vi "Execute.vi"(8 "error in (no error)":errorcluster, 10 "System In":refnum<class "abs_System.lvclass">, 11 "Node in":refnum<class "Test Numeric.lvclass">) -> (0 "error out":errorcluster, 1 "Status":T1, 2 "System Out":refnum<class "abs_System.lvclass">, 3 "Node out":refnum<class "Test Numeric.lvclass">)   [LabVIEW 2021, in "BT.lvlib" / "Test Numeric.lvclass"]
uses:
  Test Numeric.lvclass
  C:/Users/Tim/Documents/LabVIEW/2021/Behaviour Tree/Source/abs_Type Leaf/abs_Type Leaf.lvclass
  abs_Node/Status.ctl
  abs_System/abs_System.lvclass
  GitHub/LV_Abstract/Source/Abs_Types/Double Float/Abs_Double Float.lvclass
  abs_Type Leaf/abs_Type Leaf.lvclass/abs_Type Leaf.ctl
  Test Numeric.lvclass/Test Numeric.ctl
  abs_Type Leaf/Properties/Read Value Class.vi
  Properties/Read Lower Limit.vi
  Properties/Read Upper Limit.vi
  Properties/Read Limit Test Type.vi
  GitHub/LV_Abstract/Source/Functions/Compare/Support/Greater/DBL/Method.vi
  GitHub/LV_Abstract/Source/Functions/Compare/Support/Less/DBL/Method.vi
  GitHub/LV_Abstract/Source/Functions/Compare/Support/Greater Equal/DBL/Method.vi
  GitHub/LV_Abstract/Source/Functions/Compare/Support/Less Equal/DBL/Method.vi
  GitHub/LV_Abstract/Source/Functions/Logic/Support/AND/Bool/Method.vi
  GitHub/LV_Abstract/Source/Functions/Logic/Support/OR/Bool/Method.vi
  GitHub/LV_Abstract/Source/Abs_Types/Type/Abs_Type.lvclass
  GitHub/LV_Abstract/Source/Abs_Types/Numeric/Abs_Numeric.lvclass
  abs_Type Leaf/abs_Type Leaf.lvclass
  GitHub/LV_Abstract/Source/Abs_Types/Boolean/Abs_Boolean.lvclass
  GitHub/LV_Abstract/Source/Functions/Compare/Support/Equal/DBL/Method.vi
  GitHub/LV_Abstract/Source/Functions/Compare/Support/Not Equal/DBL/Method.vi
  abs_Node/abs_Node.lvclass
  GitHub/LV_Abstract/Source/Functions/Compare/Support/Greater/DBL/Greater_DBL.lvclass
  GitHub/LV_Abstract/Source/Functions/Compare/Support/Less/DBL/Less_DBL.lvclass
  GitHub/LV_Abstract/Source/Functions/Compare/Support/Greater Equal/DBL/Greater Equal_DBL.lvclass
  GitHub/LV_Abstract/Source/Functions/Compare/Support/Less Equal/DBL/Less Equal_DBL.lvclass
  GitHub/LV_Abstract/Source/Functions/Logic/Support/AND/Bool/AND_Bool.lvclass
  GitHub/LV_Abstract/Source/Functions/Logic/Support/OR/Bool/OR_Bool.lvclass
  GitHub/LV_Abstract/Source/Functions/Conversion/Support/DBL/ConvertTo_DBL.lvclass
  C:/Users/Tim/Documents/GitHub/LV_Abstract/Source/Abs_Types/Double Float/Abs_Double Float.lvclass
  C:/Users/Tim/Documents/GitHub/LV_Abstract/Source/Abs_Types/Floating Point/Abs_Floating Point.lvclass
  C:/Users/Tim/Documents/GitHub/LV_Abstract/Source/Abs_Types/Numeric/Abs_Numeric.lvclass
  C:/Users/Tim/Documents/GitHub/LV_Abstract/Source/Abs_Types/Value/Abs_Value.lvclass
  C:/Users/Tim/Documents/GitHub/LV_Abstract/Source/Abs_Types/Type/Abs_Type.lvclass
  C:/Users/Tim/Documents/GitHub/LV_Abstract/Source/Functions/Conversion/Support/DBL/ConvertTo_DBL.lvclass
  GitHub/LV_Abstract/Source/Functions/Compare/Support/Equal/DBL/Equal_DBL.lvclass
  GitHub/LV_Abstract/Source/Functions/Compare/Support/Not Equal/DBL/Not Equal_DBL.lvclass
  GitHub/LV_Abstract/Source/Functions/Math/Support/Add/DBL/Method.vi
  GitHub/LV_Abstract/Source/Functions/Math/Support/Add/DBL/Add_DBL.lvclass
  GitHub/LV_Abstract/Source/Functions/Math/Support/Subtract/DBL/Method.vi
  GitHub/LV_Abstract/Source/Functions/Math/Support/Subtract/DBL/Subtract_DBL.lvclass
  GitHub/LV_Abstract/Source/Functions/Conversion/Support/DBL/Method.vi
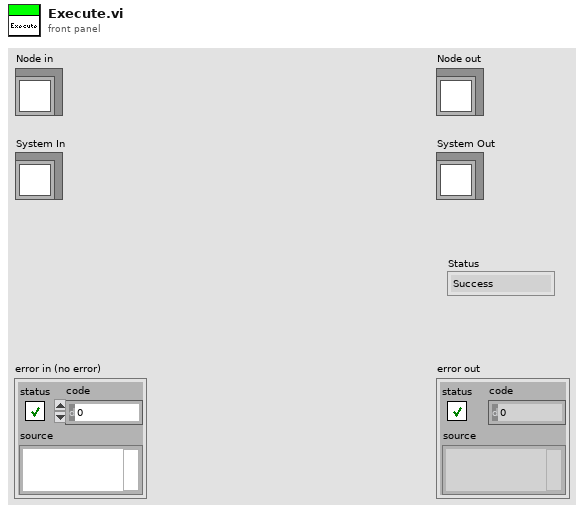
[diagram p1: front panel]
types:
  T1 = typedef "BT.lvlib/abs_Node.lvclass/Status.ctl" = enum16{"Success", "Failure", "Running"}
  T2 = typedef "BT.lvlib/Limit Test Type.ctl" = enum16{"x == Lo", "x != Lo", "x > Lo", "x < Lo", "x >= Lo", "x <= Lo", "Lo > x < Hi", "Lo >= x <= Hi", "Lo >= x < Hi", "Lo > x <= Hi", "Lo < x > Hi", "Lo <= x >= Hi", "Lo <= x > Hi", "Lo < x >= Hi", "x == Lo +/- Hi"}
  T3 = typedef "Subtract_DBL.lvclass/Abs Type.ctl" = refnum<class "Abs_Double Float.lvclass">
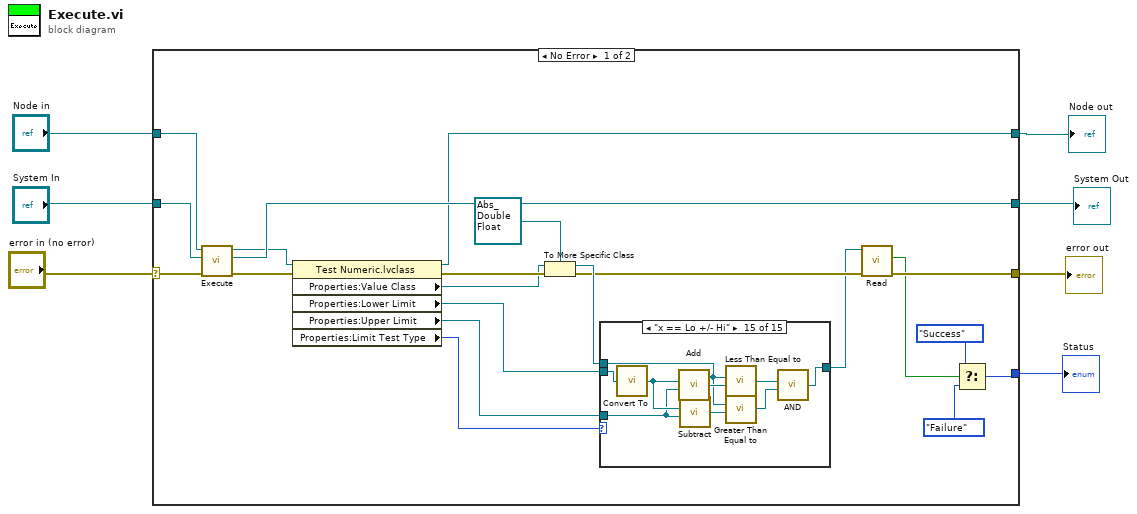
[diagram p0: block diagram]
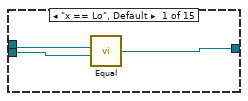
[diagram p2: hidden frame]
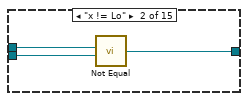
[diagram p3: hidden frame]
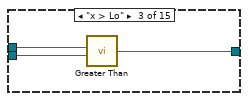
[diagram p4: hidden frame]
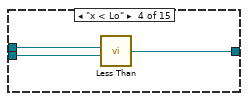
[diagram p5: hidden frame]
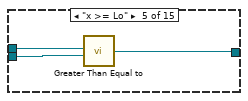
[diagram p6: hidden frame]
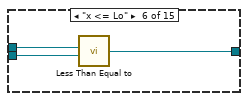
[diagram p7: hidden frame]
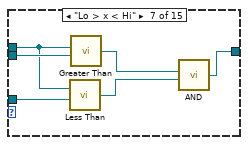
[diagram p8: hidden frame]
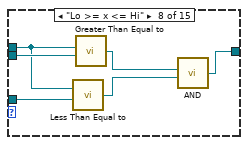
[diagram p9: hidden frame]
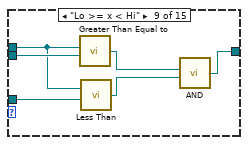
[diagram p10: hidden frame]
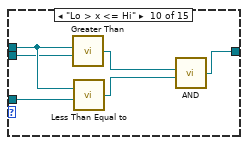
[diagram p11: hidden frame]
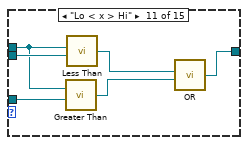
[diagram p12: hidden frame]
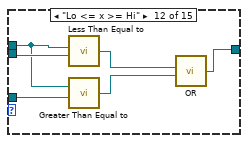
[diagram p13: hidden frame]
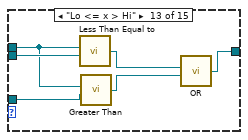
[diagram p14: hidden frame]
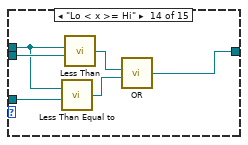
[diagram p15: hidden frame]
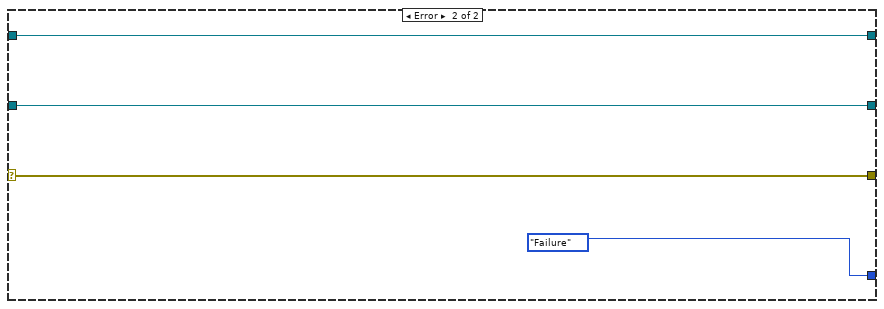
[diagram p16: hidden frame]
diagram:
  n1 = case shown="No Error" "error in (no error)" {
    selector: "error in (no error)" -> [w27 w105]
    tunnel: [w28 w106] -> w4
    tunnel: "System In" -> [w26 w106]
    tunnel: "Node in" -> [w25 w107]
    tunnel: [w9 w105] -> w7
    tunnel: [w22 w107] -> w3
    tunnel: [w19 Status."Failure" ("Status")] -> w1
    frame No Error {
      n2 = call-parent "Execute.vi"("error in (no error)"=w27, "System In"=w26, "Node in"=w25) -> ("error out"=w24:errorcluster, "System Out"=w28:refnum<class "abs_System.lvclass">, "Node out"=w23:refnum<class "Test Numeric.lvclass">)  [unwired: 5 in, 1 out]
      n3 = property class="Test Numeric.lvclass"(reference=w23, error in=w24) -> (reference out=w22:refnum<class "Test Numeric.lvclass">, error out=w15:errorcluster, "Properties:Value Class"=w13:refnum<class "Abs_Type.lvclass">, "Properties:Lower Limit"=w18:refnum<class "Abs_Numeric.lvclass">, "Properties:Upper Limit"=w16:refnum<class "Abs_Numeric.lvclass">, "Properties:Limit Test Type"=w17:T2)
      n4 = To More Specific Class(target class=refnum<class "Abs_Double Float.lvclass"> refnum ("Abs_Double Float.lvclass"), reference=w13, error in=w15) -> (specific class reference=w12:refnum<class "Abs_Double Float.lvclass">, error out=w11:errorcluster)
      n5 = case shown="\"x == Lo +/- Hi\"" w17 {
        tunnel: w12 -> [w31 w33 w37 w40 w43 w46 w51 w57 w63 w69 w73 w81 w86 w92 w99]
        tunnel: w18 -> [w30 w34 w36 w39 w42 w45 w52 w58 w64 w68 w75 w82 w88 w93 w103]
        tunnel: [w29 w32 w35 w38 w41 w44 w47 w53 w59 w65 w76 w77 w83 w89 w95] -> w10
        tunnel: w16 -> [_ _ _ _ _ _ w50 w56 w62 w70 w74 w80 w87 w94 w101]
        frame "x == Lo", Default {
          n6 = call-poly "Equal.vi"("Value B"=w30, "Value A"=w31) -> ("Result"=w29:refnum<class "Abs_Boolean.lvclass">)  [unwired: 4 in]
        }
        frame "x != Lo" {
          n7 = call-poly "Not Equal.vi"("Value B"=w34, "Value A"=w33) -> ("Result"=w32:refnum<class "Abs_Boolean.lvclass">)  [unwired: 4 in]
        }
        frame "x > Lo" {
          n8 = call-poly "Greater Than.vi"("Value B"=w36, "Value A"=w37) -> ("Result"=w35:refnum<class "Abs_Boolean.lvclass">)  [unwired: 4 in]
        }
        frame "x < Lo" {
          n9 = call-poly "Less Than.vi"("Value B"=w39, "Value A"=w40) -> ("Result"=w38:refnum<class "Abs_Boolean.lvclass">)  [unwired: 4 in]
        }
        frame "x >= Lo" {
          n10 = call-poly "Greater Than Equal to.vi"("Value B"=w42, "Value A"=w43) -> ("Result"=w41:refnum<class "Abs_Boolean.lvclass">)  [unwired: 4 in]
        }
        frame "x <= Lo" {
          n11 = call-poly "Less Than Equal to.vi"("Value B"=w45, "Value A"=w46) -> ("Result"=w44:refnum<class "Abs_Boolean.lvclass">)  [unwired: 4 in]
        }
        frame "Lo > x < Hi" {
          n12 = call-poly "Less Than.vi"("Value B"=w50, "Value A"=w51) -> ("Result"=w48:refnum<class "Abs_Boolean.lvclass">)  [unwired: 4 in]
          n13 = call-poly "Greater Than.vi"("Value B"=w52, "Value A"=w51) -> ("Result"=w49:refnum<class "Abs_Boolean.lvclass">)  [unwired: 4 in]
          n14 = call-poly "AND.vi"("B"=w48, "A"=w49) -> ("Result"=w47:refnum<class "Abs_Boolean.lvclass">)  [unwired: 4 in]
        }
        frame "Lo >= x <= Hi" {
          n15 = call-poly "Less Than Equal to.vi"("Value B"=w56, "Value A"=w57) -> ("Result"=w54:refnum<class "Abs_Boolean.lvclass">)  [unwired: 4 in]
          n16 = call-poly "Greater Than Equal to.vi"("Value B"=w58, "Value A"=w57) -> ("Result"=w55:refnum<class "Abs_Boolean.lvclass">)  [unwired: 4 in]
          n17 = call-poly "AND.vi"("B"=w54, "A"=w55) -> ("Result"=w53:refnum<class "Abs_Boolean.lvclass">)  [unwired: 4 in]
        }
        frame "Lo >= x < Hi" {
          n18 = call-poly "Greater Than Equal to.vi"("Value B"=w64, "Value A"=w63) -> ("Result"=w60:refnum<class "Abs_Boolean.lvclass">)  [unwired: 4 in]
          n19 = call-poly "Less Than.vi"("Value B"=w62, "Value A"=w63) -> ("Result"=w61:refnum<class "Abs_Boolean.lvclass">)  [unwired: 4 in]
          n20 = call-poly "AND.vi"("B"=w61, "A"=w60) -> ("Result"=w59:refnum<class "Abs_Boolean.lvclass">)  [unwired: 4 in]
        }
        frame "Lo > x <= Hi" {
          n21 = call-poly "Greater Than.vi"("Value B"=w68, "Value A"=w69) -> ("Result"=w67:refnum<class "Abs_Boolean.lvclass">)  [unwired: 4 in]
          n22 = call-poly "Less Than Equal to.vi"("Value B"=w70, "Value A"=w69) -> ("Result"=w66:refnum<class "Abs_Boolean.lvclass">)  [unwired: 4 in]
          n23 = call-poly "AND.vi"("B"=w66, "A"=w67) -> ("Result"=w65:refnum<class "Abs_Boolean.lvclass">)  [unwired: 4 in]
        }
        frame "Lo < x > Hi" {
          n24 = call-poly "Greater Than.vi"("Value B"=w74, "Value A"=w73) -> ("Result"=w71:refnum<class "Abs_Boolean.lvclass">)  [unwired: 4 in]
          n25 = call-poly "Less Than.vi"("Value B"=w75, "Value A"=w73) -> ("Result"=w72:refnum<class "Abs_Boolean.lvclass">)  [unwired: 4 in]
          n26 = call-poly "OR.vi"("B"=w71, "A"=w72) -> ("Result"=w76:refnum<class "Abs_Boolean.lvclass">)  [unwired: 4 in]
        }
        frame "Lo <= x >= Hi" {
          n27 = call-poly "Less Than Equal to.vi"("Value B"=w82, "Value A"=w81) -> ("Result"=w78:refnum<class "Abs_Boolean.lvclass">)  [unwired: 4 in]
          n28 = call-poly "Greater Than Equal to.vi"("Value B"=w80, "Value A"=w81) -> ("Result"=w79:refnum<class "Abs_Boolean.lvclass">)  [unwired: 4 in]
          n29 = call-poly "OR.vi"("B"=w79, "A"=w78) -> ("Result"=w77:refnum<class "Abs_Boolean.lvclass">)  [unwired: 4 in]
        }
        frame "Lo <= x > Hi" {
          n30 = call-poly "Less Than Equal to.vi"("Value B"=w88, "Value A"=w86) -> ("Result"=w85:refnum<class "Abs_Boolean.lvclass">)  [unwired: 4 in]
          n31 = call-poly "Greater Than.vi"("Value B"=w87, "Value A"=w86) -> ("Result"=w84:refnum<class "Abs_Boolean.lvclass">)  [unwired: 4 in]
          n32 = call-poly "OR.vi"("B"=w84, "A"=w85) -> ("Result"=w83:refnum<class "Abs_Boolean.lvclass">)  [unwired: 4 in]
        }
        frame "Lo < x >= Hi" {
          n33 = call-poly "Less Than Equal to.vi"("Value B"=w94, "Value A"=w92) -> ("Result"=w90:refnum<class "Abs_Boolean.lvclass">)  [unwired: 4 in]
          n34 = call-poly "Less Than.vi"("Value B"=w93, "Value A"=w92) -> ("Result"=w91:refnum<class "Abs_Boolean.lvclass">)  [unwired: 4 in]
          n35 = call-poly "OR.vi"("B"=w90, "A"=w91) -> ("Result"=w89:refnum<class "Abs_Boolean.lvclass">)  [unwired: 4 in]
        }
        frame "x == Lo +/- Hi" {
          n36 = call-poly "Convert To.vi"("Value"=w103) -> ("Result"=w102:refnum<class "ConvertTo_DBL.lvclass">)  [unwired: 4 in]
          n37 = call-poly "Add.vi"("Abs_Types.lvlib:Numeric.lvclass"=w101, "Input A"=w102) -> ("Result"=w100:refnum<class "Abs_Double Float.lvclass">)  [unwired: 4 in]
          n38 = call-poly "Subtract.vi"("Input B"=w101, "Input A"=w102) -> ("Result"=w98:T3)  [unwired: 4 in]
          n39 = call-poly "Less Than Equal to.vi"("Value B"=w100, "Value A"=w99) -> ("Result"=w97:refnum<class "Abs_Boolean.lvclass">)  [unwired: 4 in]
          n40 = call-poly "Greater Than Equal to.vi"("Value B"=w98, "Value A"=w99) -> ("Result"=w96:refnum<class "Abs_Boolean.lvclass">)  [unwired: 4 in]
          n41 = call-poly "AND.vi"("B"=w96, "A"=w97) -> ("Result"=w95:refnum<class "Abs_Boolean.lvclass">)  [unwired: 4 in]
        }
      }
      n42 = call-dynamic "Read.vi"("error in (no error)"=w11, "Boolean in"=w10) -> ("error out"=w9:errorcluster, "Boolean"=w8:bool)  [unwired: 7 in, 1 out]
      n43 = Select(t=Status."Success" ("Status"), s=w8, f=Status."Failure") -> (s? t:f=w19:T1)
    }
    frame Error {
    }
  }
  "error out" <- w7
  "Node out" <- w3
  "Status" <- w1
  "System Out" <- w4
